vi "Create File with Folder.vi"() -> ()   [LabVIEW 2021]
panel:
  in  "Name or path File 2":string
  in  "Name or path":string
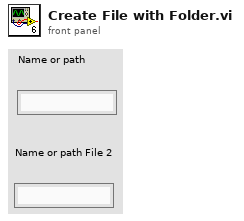
[diagram p1: front panel]
types:
  T1 = enum16{"open", "replace", "create", "open or create", "replace or create", "replace or create with confirmation"}
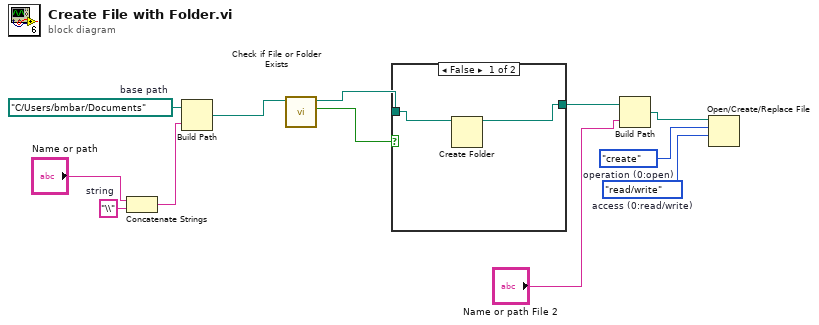
[diagram p0: block diagram]
diagram:
  w4 = "\\"  # string
  w5 = enum16{"read/write", "read-only", "write-only"}."read/write"  # access (0:read/write)
  w6 = T1."create"  # operation (0:open)
  w11 = path "C:/Users/bmbar/Documents"  # base path
  n1 = Concatenate Strings "Concatenate Strings"("Name or path", w4) -> (w2:string)
  n2 = Build Path(base path=w11, name or relative path=w2) -> (appended path=w12:path)
  n3 = call <vilib>:"Check if File or Folder Exists.vi"("path"=w12) -> ("file or folder exists?"=w9:bool, "dup path"=w10:path)  [unwired: 8 in, 1 out]
  n4 = case shown="False" w9 {
    tunnel: w10 -> [w14 w15]
    tunnel: [w13 w15] -> w8
    frame False {
      n5 = Create Folder(path (use dialog)=w14) -> (created path=w13:path)  [unwired: 2 in, 2 out]
    }
    frame True {
    }
  }
  n6 = Build Path(base path=w8, name or relative path="Name or path File 2") -> (appended path=w7:path)
  n7 = Open/Create/Replace File(file path (use dialog)=w7, operation (0:open)=w6, access (0:read/write)=w5) -> ()  [unwired: 3 in, 3 out]
